vi "class_data.vi"() -> ()   [LabVIEW 2010, in "GenericToplevelComponent.lvclass"]
uses:
  GenericToplevelComponent.lvclass
panel:
  in  "loaded components":string[](array[string])
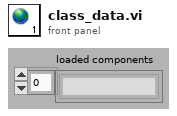
[diagram p1: front panel]
diagram:
